vi "Configure Integration.vi"(0 "VISA resource name":refnum<visa-resource-name>, 1 "Integration Mode (0: Normal)":i32(ring) items=["Normal", "Continuous"], 5 "Integration Time Hour (0)":i32 min=0 max=10000, 7 "Integration Time Minute (0)":i32 min=0 max=59, 9 "Integration Time Second (0)":i32 min=0 max=59, 11 "error in (no error)":errorcluster) -> (4 "VISA resource name out":refnum<visa-resource-name>, 15 "error out":errorcluster)   [LabVIEW 2016, in "Yokogawa WT300 Series.lvlib"]
doc: "Configures the integrated power features."
uses:
  Yokogawa WT300 Series.lvlib
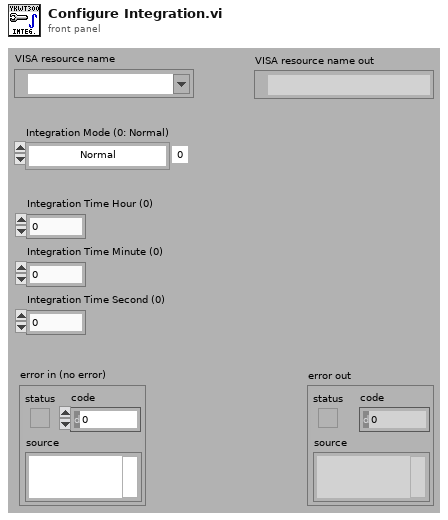
[diagram p1: front panel]
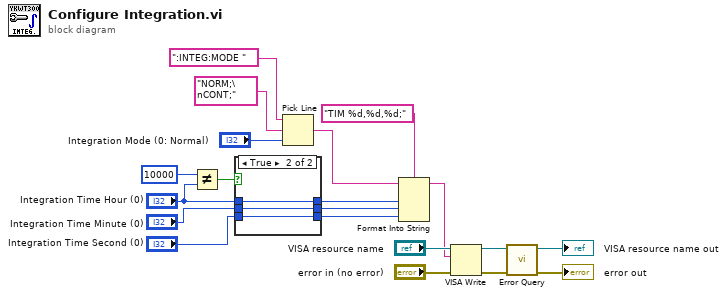
[diagram p0: block diagram]
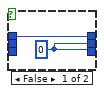
[diagram p2: hidden frame]
diagram:
  n1 = Not Equal?(x=10000, y="Integration Time Hour (0)") -> (x != y?=w8:bool)
  n2 = case shown="True" w8 {
    tunnel: "Integration Time Hour (0)" -> [w22 w25]
    tunnel: [w22 w25] -> w5
    tunnel: "Integration Time Minute (0)" -> [_ w24]
    tunnel: [w21 w24] -> w3
    tunnel: "Integration Time Second (0)" -> [_ w23]
    tunnel: [w21 w23] -> w1
    frame False {
      w21 = 0
    }
    frame True {
    }
  }
  n3 = Pick Line ("ライン選択")(string ("")=":INTEG:MODE ", multi-line string="NORM;\nCONT;" ("¡s¶ñ"), line index="Integration Mode (0: Normal)") -> (output string=w10:string)
  n4 = Format Into String(format string="TIM %d,%d,%d;" ("Œ`Ž®•¶Žš—ñ"), initial string=w10, w5, w3, w1) -> (resulting string=w11:string)  [unwired: 1 in, 1 out]
  n5 = VISA Write ("VISA書き込み")(VISA resource name="VISA resource name", write buffer=w11, error in (no error)="error in (no error)") -> (VISA resource name out=w20:refnum<visa-resource-name>, error out=w19:errorcluster)  [unwired: 1 out]
  n6 = call "Error Query.vi"("error in (no error)"=w19, "VISA resource name"=w20) -> ("error out"=→"error out":errorcluster, "VISA resource name out"=→"VISA resource name out":refnum<visa-resource-name>)  [unwired: 6 in, 2 out]
